vi "RCV Test_ks5080A_w-Beam.vi"(0 "Semiconductor Module Context":T2, 1 "Meas Type":T6, 2 "Test Information":T5={"Exp Name"="Cold Switching", "Lot"="0233A", "Wafer"="15", "Die Type"="L22", "Die X "="6", "Die Y"="8", "Exp"="1", "Die X_Y"="8"}, 3 "# of Cycles":string, 5 "Sweep Settings":T3={"Start"=0.0, "Stop"=1.0, "Step"=0.0}, 7 "Test_Pins":T4={"RF_Pins"=["RF1", "RF2"], "Contact_Meas_Pins"=["RF1"], "Contact_Source_Pins"=["RF1"], "Sweep_Bias_Pins"=[]}, 9 "error in (no error)":errorcluster, 12 "Averaging Count":i32=3, 13 "Plots FilePath":path=path "C:/Users/DalLab/Desktop/Test Data/Plots") -> (4 "ks5080A_Meaurements":T7, 15 "error out":errorcluster)   [LabVIEW 2013]
doc: "Initiates and fetches niVNA S11 measurements and converts it to a capacitance measurement."
uses:
  <vilib>/NI_TestStand_SemiconductorModule/NI_TestStand_Semiconductor_Module.lvlibp/PinMap/General/SemiconductorModuleContext.ctl
  Controls/Sweep Settings.ctl
  Controls/Test_Pins.ctl
  Controls/Test Information.ctl
  Controls/Meas Type.ctl
  Controls/ks5080A_Measurements.ctl
  <vilib>/NI_TestStand_SemiconductorModule/NI_TestStand_Semiconductor_Module.lvlibp
panel:
  in  "Tab Control":enum32{"Graphs", "Controls and Indicators"}(tab)
  out "Wafer":string
  out "Die Type":string
  out "Measurement":string
  out "Die X_Y":string
  out "Graph Cluster":T1
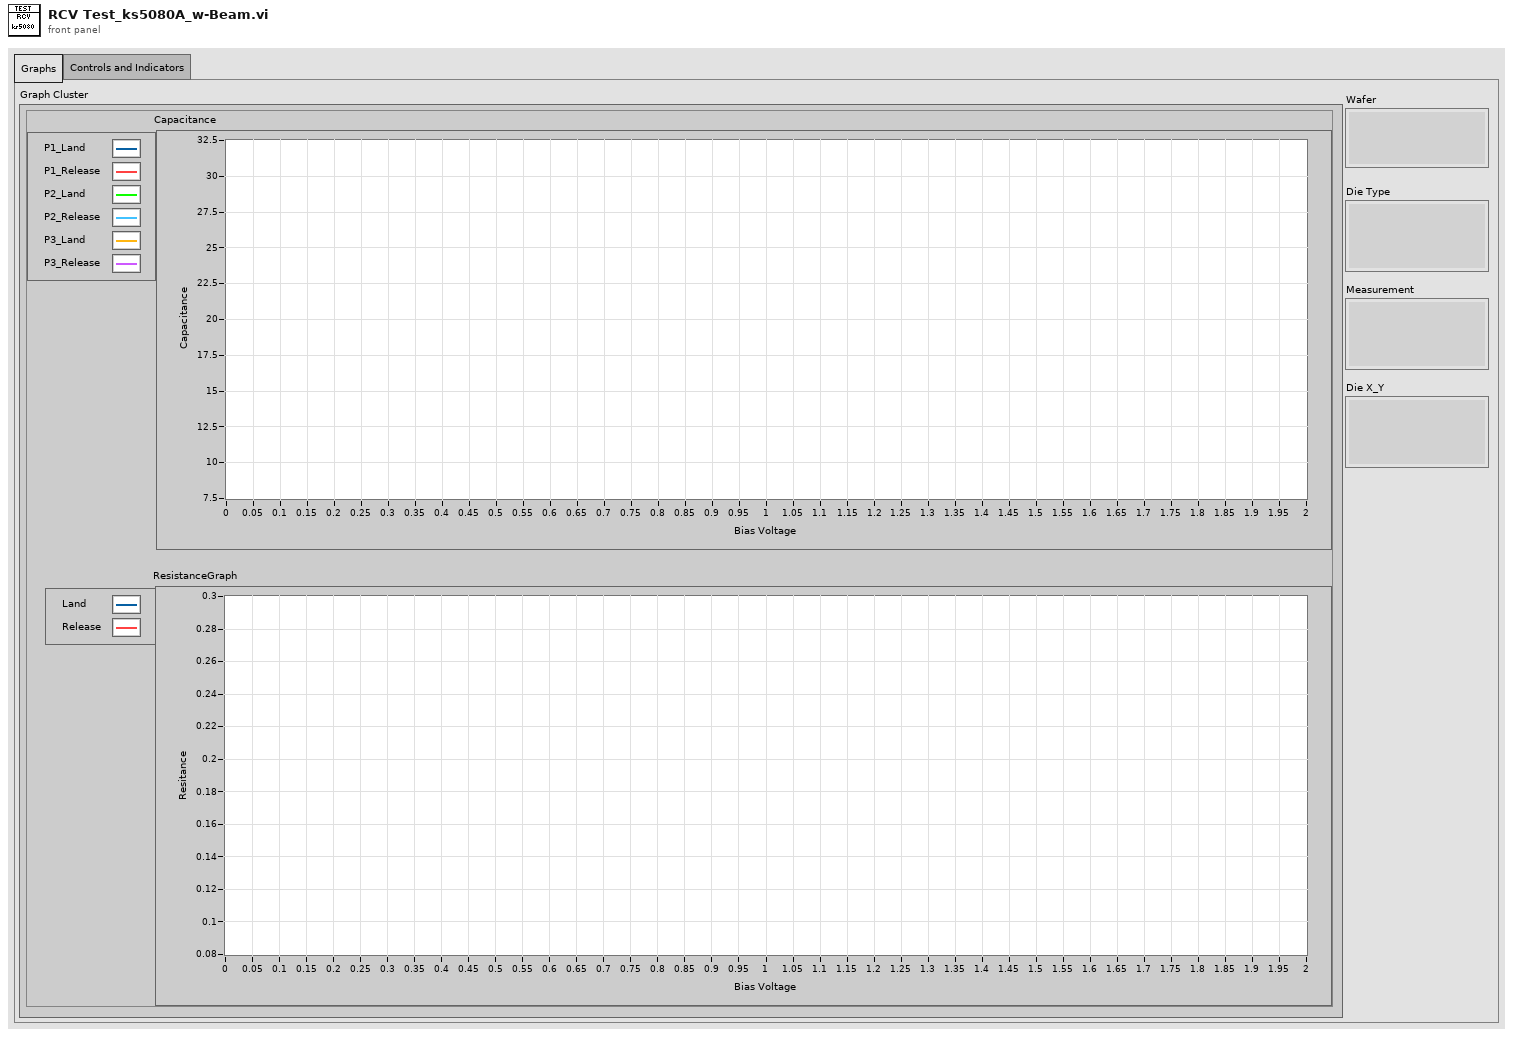
[diagram p1: front panel]
types:
  T1 = cluster{"ResistanceGraph":cluster{dbl[], dbl[]}[], "Capacitance":cluster{dbl[], dbl[]}[]}
  T2 = typedef "NI_TestStand_Semiconductor_Module.lvlibp/SemiconductorModuleContext.ctl" = refnum<k7>
  T3 = typedef "Sweep Settings.ctl" = cluster{"Start":dbl, "Stop":dbl, "Step":dbl}
  T4 = typedef "Test_Pins.ctl" = cluster{"RF_Pins":string[], "Contact_Meas_Pins":string[], "Contact_Source_Pins":string[], "Sweep_Bias_Pins":string[]}
  T5 = typedef "Test Information.ctl" = cluster{"Exp Name":string, "Lot":string, "Wafer":string, "Die Type":string, "Die X ":string, "Die Y":string, "Exp":string, "Die X_Y":string}
  T6 = typedef "Meas Type.ctl" = enum16{"Floor", "Roof", "Buckling", "Charge Transfer"}
  T7 = typedef "ks5080A_Measurements.ctl" = cluster{"Bias_Sweep_Setting":dbl[], "Bias_voltage measurements":dbl[], "Bias_current measurements":dbl[], "P1_Capacitance":dbl[], "P2_Capacitance":dbl[], "DMM_Measurement_V":dbl[], "Contact_Source Current measurements":dbl[], "Contact_Sink Current measurements":dbl[], "Calculated_Resistance":dbl[], "P3_Capacitance":dbl[], "Port 1_S_parm":string[], "Port 2_S_parm":string[], "Port 3_S_parm":string[]}
  T8 = typedef "ENA_Marker Measurements.ctl" = cluster{"Port 1 Capacitance":dbl[], "Port 2 Capacitance":dbl[], "Port 3 Capacitance":dbl[], "Port 1_S_parm":string[], "Port 2_S_parm":string[], "Port 3_S_parm":string[]}
  T9 = typedef "imagedata.ctl" = cluster{"image type":i32, "image depth":i32, "image":u8[], "mask":u8[], "colors":u32[], "Rectangle":cluster{"left":i16, "top":i16, "right":i16, "bottom":i16}}
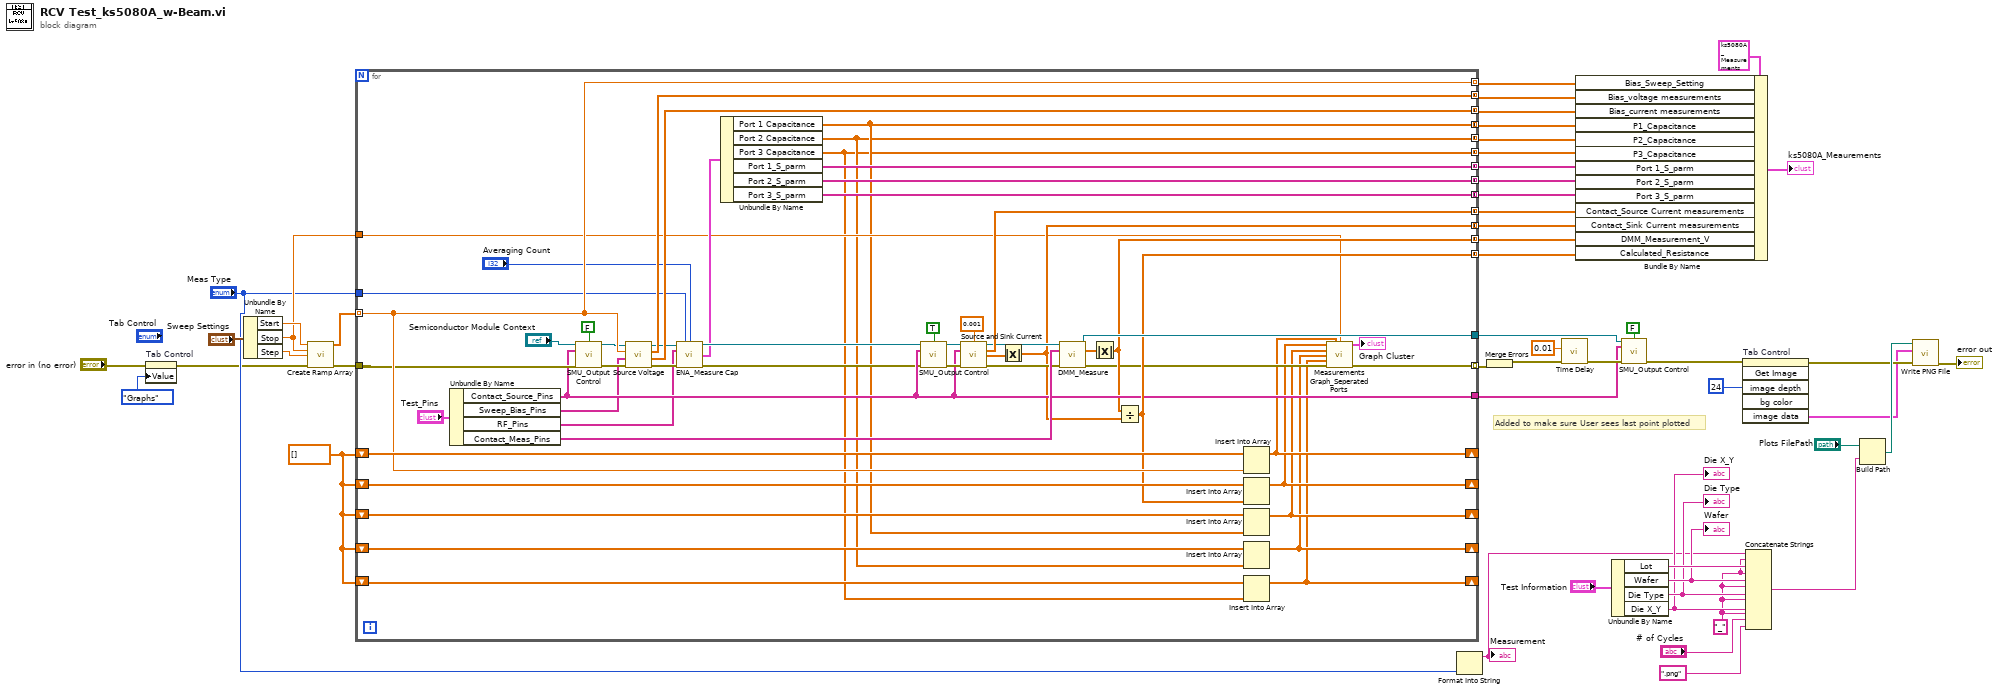
[diagram p0: block diagram]
diagram:
  w4 = "_"
  w1 = dbl[] []
  # "Added to make sure User sees last point plotted"
  n1 = property on="Tab Control" class="TabCtl (strict)"(error in="error in (no error)", "Value"=enum32{"Graphs", "Controls and Indicators"}."Graphs" ("Tab Control")) -> (error out=w5:errorcluster)  [unwired: 1 in, 1 out]
  n2 = Unbundle By Name("Sweep Settings") -> ("Start"=w46:dbl, "Stop"=w44:dbl, "Step"=w45:dbl)
  n3 = call "Create Ramp Array.vi"("Start"=w46, "Stop"=w44, "Step"=w45, "Error In"=w5) -> ("Ramp Pattern"=w50:dbl[], "Error Out"=w48:errorcluster)  [unwired: 10 in]
  n4 = for {
    tunnel: w50 -> [w96] mode=indexing
    tunnel: [w103] -> w36 mode=concatenating
    tunnel: [w102] -> w35 mode=concatenating
    tunnel: [w69] -> w32 mode=concatenating
    tunnel: [w63] -> w49 mode=indexing
    tunnel: w48 -> [w95]
    tunnel: w44 -> [w62]
    shift-right: [w56] -> _
    shift-left: w1 -> [w99]
    shift-right: [w55] -> _
    shift-left: w1 -> [w98]
    shift-right: [w54] -> _
    shift-left: w1 -> [w97]
    tunnel: [w96] -> w37 mode=indexing
    tunnel: [w88] -> w39
    tunnel: [w81] -> w38
    tunnel: [w87] -> w34 mode=concatenating
    tunnel: [w66] -> w33 mode=concatenating
    tunnel: [w86] -> w31 mode=concatenating
    tunnel: [w59] -> w19 mode=concatenating
    tunnel: [w58] -> w18 mode=concatenating
    tunnel: [w57] -> w17 mode=concatenating
    tunnel: [w72] -> w16 mode=concatenating
    tunnel: [w71] -> w15 mode=concatenating
    tunnel: [w70] -> w14 mode=concatenating
    tunnel: "Meas Type" -> [w65]
    shift-right: [w53] -> _
    shift-left: w1 -> [w61]
    shift-right: [w52] -> _
    shift-left: w1 -> [w60]
    n5 = Unbundle By Name("Test_Pins") -> ("Contact_Source_Pins"=w81:string[], "Sweep_Bias_Pins"=w80:string[], "RF_Pins"=w77:string[], "Contact_Meas_Pins"=w100:string[])
    n6 = call "SMU_Output Control.vi"("Semiconductor Module Context"="Semiconductor Module Context", "output enabled?"=FALSE, "Pins"=w81, "error in (no error)"=w95) -> ("Semiconductor Module Context Out"=w92:T2, "error out"=w94:errorcluster)  [unwired: 10 in]
    n7 = call "Source Voltage.vi"("error in (no error)"=w94, "Pins"=w80, "voltage level"=w96, "Semiconductor Module Context"=w92) -> ("error out"=w79:errorcluster, "current measurements"=w102:dbl[], "voltage measurements"=w103:dbl[], "Semiconductor Module Context Out"=w76:T2)  [unwired: 4 in]
    n8 = call "ENA_Measure Cap.vi"("Semiconductor Module Context"=w76, "Meas Type"=w65, "Averaging Count"="Averaging Count", "Pins"=w77, "error in (no error)"=w79) -> ("Semiconductor Module Context Out"=w75:T2, "Marker Measurements"=w73:T8, "error out"=w78:errorcluster)  [unwired: 8 in]
    n9 = Unbundle By Name(w73) -> ("Port 1 Capacitance"=w59:dbl[], "Port 2 Capacitance"=w58:dbl[], "Port 3 Capacitance"=w57:dbl[], "Port 1_S_parm"=w72:string[], "Port 2_S_parm"=w71:string[], "Port 3_S_parm"=w70:string[])
    n10 = call "SMU_Output Control.vi"("Semiconductor Module Context"=w75, "output enabled?"=TRUE, "Pins"=w81, "error in (no error)"=w78) -> ("Semiconductor Module Context Out"=w82:T2, "error out"=w83:errorcluster)  [unwired: 10 in]
    n11 = call "Source and Sink Current.vi"("Semiconductor Module Context"=w82, "Current level"=0.001, "Pins"=w81, "error in (no error)"=w83) -> ("Semiconductor Module Context Out"=w84:T2, "Source Current measurements"=w87:dbl[], "Sink Current measurements"=w67:dbl[], "error out"=w85:errorcluster)  [unwired: 8 in]
    n12 = Absolute Value(x=w67) -> (abs(x)=w66:dbl[])
    n13 = call "DMM_Measure.vi"("Semiconductor Module Context"=w84, "Pins"=w100, "Error In"=w85) -> ("Semiconductor Module Context Out"=w88:T2, "Measurement"=w68:dbl[], "Error Out"=w64:errorcluster)  [unwired: 10 in]
    n14 = Absolute Value(x=w68) -> (abs(x)=w69:dbl[])
    n15 = Divide(x=w69, y=w66) -> (x/y=w86:dbl[])
    n16 = Insert Into Array(array=w99, new element=w96) -> (w56:dbl[])  [unwired: 1 in]
    n17 = Insert Into Array(array=w98, new element=w86) -> (w55:dbl[])  [unwired: 1 in]
    n18 = Insert Into Array(array=w97, new element=w59) -> (w54:dbl[])  [unwired: 1 in]
    n19 = Insert Into Array(array=w61, new element=w58) -> (w53:dbl[])  [unwired: 1 in]
    n20 = Insert Into Array(array=w60, new element=w57) -> (w52:dbl[])  [unwired: 1 in]
    n21 = call "Measurements Graph_Seperated Ports.vi"("Resitance"=w55, "Bias Voltage"=w56, "Stop_V"=w62, "P1"=w54, "P2"=w53, "P3"=w52, "Error In"=w64) -> ("Graph Cluster"=→"Graph Cluster":T1, "Error Out"=w63:errorcluster)  [unwired: 7 in]
  }
  n22 = Format Into String("Meas Type") -> (resulting string=w13:string)  [unwired: 3 in, 1 out]
  "Measurement" <- w13
  n23 = Merge Errors(w49) -> (w42:errorcluster)
  n24 = call "Time Delay"("error in (no error)"=w42, "Delay Time (s)"=0.01) -> ("error out"=w40:errorcluster)  [unwired: 9 in]
  n25 = Bundle By Name(cluster=T7 {"Bias_Sweep_Setting"=[], "Bias_voltage measurements"=[], "Bias_current measurements"=[], "P1_Capacitance"=[], "P2_Capacitance"=[], "DMM_Measurement_V"=[], "Contact_Source Current measurements"=[], "Contact_Sink Current measurements"=[], "Calculated_Resistance"=[], "P3_Capacitance"=[], "Port 1_S_parm"=[], "Port 2_S_parm"=[], "Port 3_S_parm"=[]} ("ks5080A_Meaurements 2"), "Bias_Sweep_Setting"=w37, "Bias_voltage measurements"=w36, "Bias_current measurements"=w35, "P1_Capacitance"=w19, "P2_Capacitance"=w18, "P3_Capacitance"=w17, "Port 1_S_parm"=w16, "Port 2_S_parm"=w15, "Port 3_S_parm"=w14, "Contact_Source Current measurements"=w34, "Contact_Sink Current measurements"=w33, "DMM_Measurement_V"=w32, "Calculated_Resistance"=w31) -> (→"ks5080A_Meaurements":T7)
  n26 = Unbundle By Name("Test Information") -> ("Lot"=w29:string, "Wafer"=w28:string, "Die Type"=w27:string, "Die X_Y"=w26:string)
  "Wafer" <- w28
  "Die Type" <- w27
  "Die X_Y" <- w26
  n27 = call "SMU_Output Control.vi"("Semiconductor Module Context"=w39, "output enabled?"=FALSE, "Pins"=w38, "error in (no error)"=w40) -> ("error out"=w11:errorcluster)  [unwired: 10 in, 1 out]
  n28 = invoke on="Tab Control" class="TabCtl (strict)" method="Get Image"(error in=w11, "image depth"=24 ("Image Depth")) -> (error out=w10:errorcluster, "image data"=w9:T9)  [unwired: 4 in, 4 out]
  n29 = Concatenate Strings(w13, w4, w29, w4, w28, w4, w27, w4, w26, w4, "# of Cycles", ".png" ("string")) -> (w25:string)
  n30 = Build Path(base path="Plots FilePath", name or relative path=w25) -> (appended path=w23:path)
  n31 = call <vilib>:"Write PNG File.vi"("error in (no error)"=w10, "image data"=w9, "path to PNG file"=w23) -> ("error out"=→"error out":errorcluster)  [unwired: 7 in, 1 out]
